vi "Calibrate Channel N.vi"(0 "EPU452 in":refnum<class "EPU452.lvclass">, 5 "Channel":T1, 7 "Function":string, 9 "Argument/s":string, 11 "error in (no error)":errorcluster) -> (4 "EPU452 out":refnum<class "EPU452.lvclass">, 8 "Response":string, 15 "error out":errorcluster)   [LabVIEW 2018, in "EPU452.lvclass"]
uses:
  EPU452.lvclass
  Controls/Channels.ctl
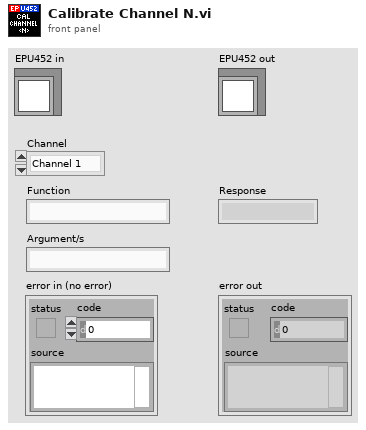
[diagram p1: front panel]
types:
  T1 = typedef "EPU452.lvclass/Channels.ctl" = enum16{"Channel 1", "Channel 2", "Channel 3", "Channel 4"}
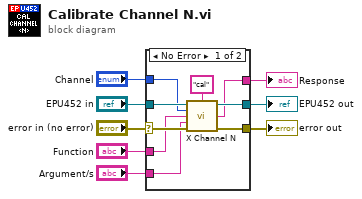
[diagram p0: block diagram]
diagram:
  n1 = case shown="No Error" "error in (no error)" {
    selector: "error in (no error)" -> [w17 w19]
    tunnel: [w14 w19] -> w7
    tunnel: [w13 w18] -> w5
    tunnel: "EPU452 in" -> [w16 w18]
    tunnel: "Channel" -> [w15 _]
    tunnel: [w12 _] -> w3
    tunnel: "Function" -> [w11 _]
    tunnel: "Argument/s" -> [w10 _]
    frame No Error {
      n2 = call "X Channel N.vi"("EPU452 in"=w16, "Operation"="cal", "Channel"=w15, "Function"=w11, "Argument/s"=w10, "error in (no error)"=w17) -> ("EPU452 out"=w13:refnum<class "EPU452.lvclass">, "Response"=w12:string, "error out"=w14:errorcluster)  [unwired: 7 in]
    }
    frame Error {
    }
  }
  "error out" <- w7
  "EPU452 out" <- w5
  "Response" <- w3
